vi "pp_trialType_toStringArray.vi"(11 "Input Trial Cluster":T1={"Trial Code"=1, "Trial Type"=enum."GO", "Trial Weight"=0, "Stim Type"=enum."FM Sweep", "Stim Dur (s)"=2.0, "Stim P1"=4.0, "Stim P2"=0.0} {"Stim P2" min=0.0; "Trial Weight" step=1; "Stim P1" min=0.0; "Stim Dur (s)" min=0.0; "Trial Code" min=1 step=1}) -> (3 "Output string array":string[](array[string]))   [LabVIEW 2013]
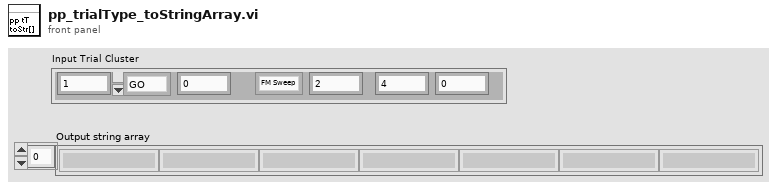
[diagram p1: front panel]
types:
  T1 = cluster{"Trial Code":u16, "Trial Type":enum16{"OFF", "GO", "NOGO", "TEST"}, "Trial Weight":u32, "Stim Type":enum16{"Pure Tone", "FM Sweep"}, "Stim Dur (s)":dbl, "Stim P1":dbl, "Stim P2":dbl}
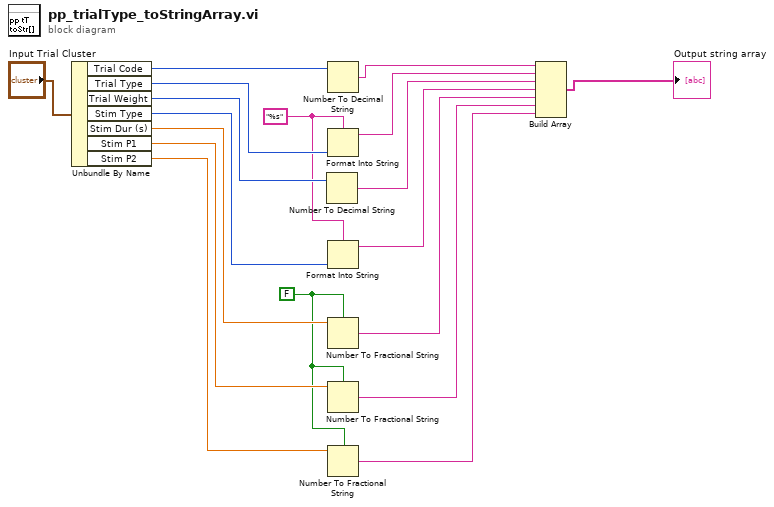
[diagram p0: block diagram]
diagram:
  w9 = FALSE ("use system decimal point (T)")
  w13 = "%s" ("format string")
  n1 = Unbundle By Name("Input Trial Cluster") -> ("Trial Code"=w16:u16, "Trial Type"=w17:enum16{"OFF", "GO", "NOGO", "TEST"}, "Trial Weight"=w15:u32, "Stim Type"=w14:enum16{"Pure Tone", "FM Sweep"}, "Stim Dur (s)"=w12:dbl, "Stim P1"=w11:dbl, "Stim P2"=w10:dbl)
  n2 = Number To Decimal String(number=w15) -> (decimal integer string=w6:string)  [unwired: 1 in]
  n3 = Number To Decimal String(number=w16) -> (decimal integer string=w8:string)  [unwired: 1 in]
  n4 = Format Into String(format string=w13, w17) -> (resulting string=w7:string)  [unwired: 2 in, 1 out]
  n5 = Format Into String(format string=w13, w14) -> (resulting string=w5:string)  [unwired: 2 in, 1 out]
  n6 = Number To Fractional String(use system decimal point (T)=w9, number=w12) -> (F-format string=w4:string)  [unwired: 2 in]
  n7 = Number To Fractional String(use system decimal point (T)=w9, number=w11) -> (F-format string=w3:string)  [unwired: 2 in]
  n8 = Number To Fractional String(use system decimal point (T)=w9, number=w10) -> (F-format string=w2:string)  [unwired: 2 in]
  n9 = Build Array(w8, w7, w6, w5, w4, w3, w2) -> (→"Output string array":string[])
